vi "NIDCPower_channel_ganging - fetch multiple.vi"(0 "Ganged Session In":T2, 9 "Count":i32, 11 "error in (no error)":errorcluster) -> (2 "Ganged Voltage Measurement":dbl[](array[numeric]), 3 "Ganged Current Measurement":dbl[](array[numeric]), 4 "Ganged Session Out":T2, 6 "voltage measurements":dbl[][](array[numeric]) format="%#_6p", 8 "current measurements":dbl[][](array[numeric]) format="%#_6p", 10 "in compliance":bool[][](array[boolean]), 14 "Measure Record dt":dbl[](array[numeric]), 15 "error out":errorcluster)   [LabVIEW 2021]
uses:
  ctl/NIDCPower_channel_ganging - ctl - ganged config.ctl
  ctl/NIDCPower_channel_ganging - ctl - channel mode.ctl
  ctl/NIDCPower_channel_ganging - ctl - ganged session.ctl
panel:
  out "Waveform Graph":dbl[](graph)
  in  "Ganged Config":T1=enum."Parallel"
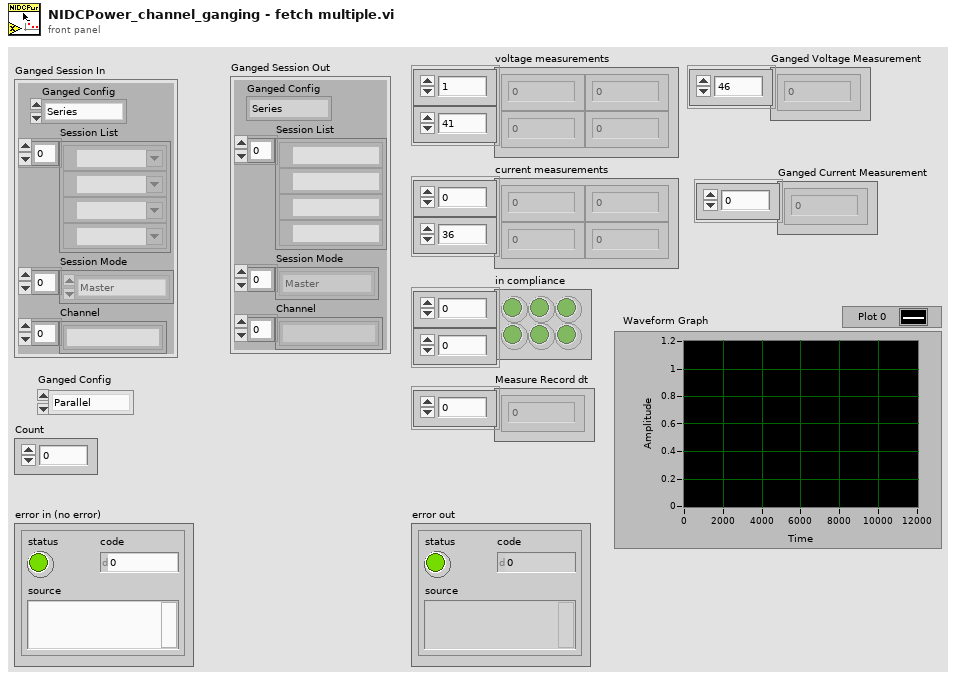
[diagram p1: front panel]
types:
  T1 = typedef "NIDCPower_channel_ganging - ctl - ganged config.ctl" = enum16{"Series", "Parallel", "Manual"}
  T2 = typedef "NIDCPower_channel_ganging - ctl - ganged session.ctl" = cluster{"Ganged Config":T1, "Session List":refnum<k15>[], "Session Mode":T3[], "Channel":string[]}
  T3 = typedef "NIDCPower_channel_ganging - ctl - channel mode.ctl" = enum16{"Master", "Slave", "Slave - Inverted"}
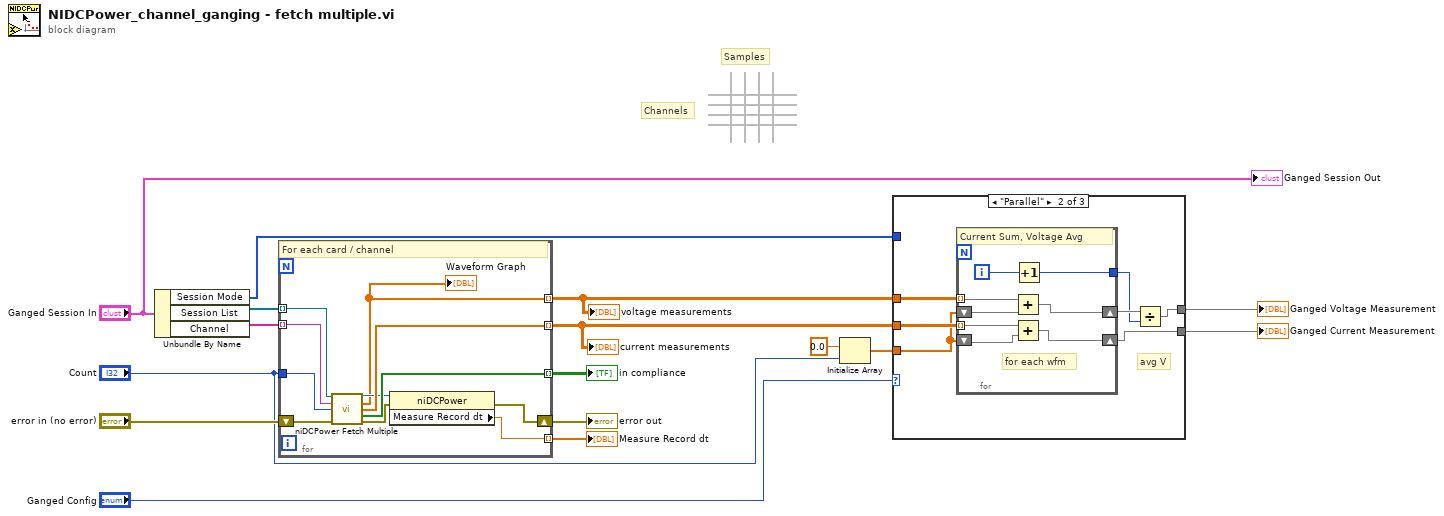
[diagram p0: block diagram]
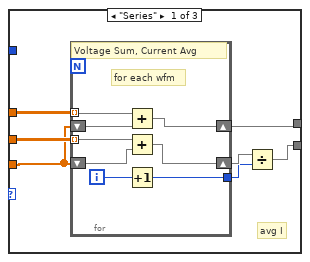
[diagram p2: hidden frame]
diagram:
  # "Channels"
  # "Samples"
  n1 = Unbundle By Name("Ganged Session In") -> ("Session Mode"=w2:T3[], "Session List"=w13:refnum<k15>[], "Channel"=w15:string[])
  n2 = for {
    tunnel: w13 -> [w26] mode=indexing
    shift-right: [w22] -> w12
    shift-left: "error in (no error)" -> [w25]
    tunnel: "Count" -> [w27]
    tunnel: w15 -> [w17] mode=indexing
    tunnel: [w18] -> w1 mode=indexing
    tunnel: [w24] -> w5 mode=indexing
    tunnel: [w23] -> w11 mode=indexing
    tunnel: [w19] -> w10 mode=indexing
    # "For each card / channel"
    n3 = call <instrlib>:"niDCPower Fetch Multiple.vi"("instrument handle"=w26, "channel name"=w17, "count (1)"=w27, "error in (no error)"=w25) -> ("instrument handle out"=w21:refnum<k15>, "voltage measurements"=w18:dbl[], "current measurements"=w24:dbl[], "in compliance"=w23:bool[], "error out"=w20:errorcluster)  [unwired: 6 in, 1 out]
    "Waveform Graph" <- w18
    n4 = property class="niDCPower"(reference=w21, error in=w20) -> (error out=w22:errorcluster, "Measure Record dt"=w19:dbl)  [unwired: 1 out]
  }
  "error out" <- w12
  "in compliance" <- w11
  "current measurements" <- w5
  "voltage measurements" <- w1
  "Measure Record dt" <- w10
  n5 = Initialize Array(0.0 ("element"), "Count") -> (w6:dbl[])
  n6 = case shown="\"Parallel\"" "Ganged Config" {
    tunnel: w5 -> [w33 w49 _]
    tunnel: [w28 w48 _] -> w4
    tunnel: [w31 w43 _] -> w3
    tunnel: w1 -> [w34 w47 _]
    tunnel: w6 -> [w32 w46 _]
    tunnel: w2 -> [_ _ _]
    frame "Series" {
      # "avg I"
      n7 = for {
        shift-right: [w40] -> w30
        shift-left: w32 -> [w42]
        tunnel: w33 -> [w41] mode=indexing
        tunnel: w34 -> [w39] mode=indexing
        shift-right: [w37] -> w31
        shift-left: w32 -> [w38]
        tunnel: [w35] -> w29
        i -> [w36]
        # "for each wfm"
        # "Voltage Sum, Current Avg"
        n8 = Add(x=w39, y=w38) -> (x+y=w37:dbl[])
        n9 = Add(x=w41, y=w42) -> (x+y=w40:dbl[])
        n10 = Increment(x=w36) -> (x+1=w35:i32)
      }
      n11 = Divide(x=w30, y=w29) -> (x/y=w28:dbl[])
    }
    frame "Parallel" {
      # "avg V"
      n12 = for {
        shift-right: [w55] -> w48
        shift-left: w46 -> [w57]
        tunnel: w49 -> [w56] mode=indexing
        tunnel: w47 -> [w54] mode=indexing
        shift-right: [w52] -> w45
        shift-left: w46 -> [w53]
        tunnel: [w50] -> w44
        i -> [w51]
        # "for each wfm"
        # "Current Sum, Voltage Avg"
        n13 = Add(x=w54, y=w53) -> (x+y=w52:dbl[])
        n14 = Add(x=w56, y=w57) -> (x+y=w55:dbl[])
        n15 = Increment(x=w51) -> (x+1=w50:i32)
      }
      n16 = Divide(x=w45, y=w44) -> (x/y=w43:dbl[])
    }
    frame "Manual" {
    }
  }
  "Ganged Current Measurement" <- w4
  "Ganged Voltage Measurement" <- w3
  "Ganged Session Out" <- "Ganged Session In"
